vi "Trigger Level.vi"(7 "Read Value? (F)":bool, 8 "error in (no error)":errorcluster, 10 "Trigger Level (2.000 V)":dbl=2.0 min=-2.0 max=2.0 step=0.001 format="%.3g", 11 "VISA resource name":refnum<visa-resource-name>) -> (0 "error out":errorcluster, 2 "Trigger Level":dbl=2.0 format="%.3g", 3 "VISA resource name out":refnum<visa-resource-name>)   [LabVIEW 2013, in "SRS SR400.lvlib"]
doc: "<B>TL { v }</B>\n\nIf v is absent, the TL command returns the gate trigger level. When v is included, the trigger level is set to v Volts where -2.000 <= v <= 2.000. The resolution is .001 V."
uses:
  <instrlib>/SRS SR400/SRS SR400.lvlib
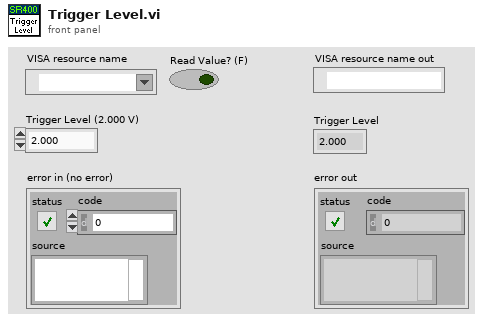
[diagram p1: front panel]
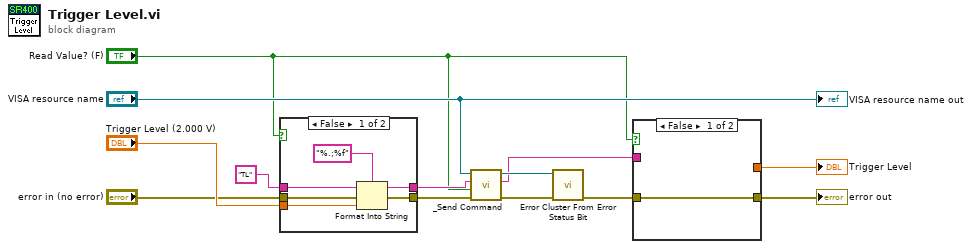
[diagram p0: block diagram]
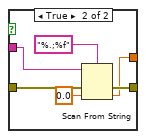
[diagram p2: hidden frame]
diagram:
  n1 = case shown="False" "Read Value? (F)" {
    tunnel: "Trigger Level (2.000 V)" -> [w19 _]
    tunnel: "error in (no error)" -> [w18 w20]
    tunnel: [w16 w21] -> w11
    tunnel: [w15 w20] -> w10
    tunnel: "TL" ("command") -> [w14 w21]
    frame False {
      n2 = Format Into String(format string="%.;%f", initial string=w14, error in=w18, w19) -> (resulting string=w16:string, error out=w15:errorcluster)
    }
    frame True {
    }
  }
  n3 = call <instrlib>:"_Send Command.vi"("error in (no error)"=w10, "Read Value? (F)"="Read Value? (F)", "Command"=w11, "VISA resource name"="VISA resource name") -> ("error out"=w7:errorcluster, "Response"=w3:string, "VISA resource name out"=w8:refnum<visa-resource-name>)  [unwired: 5 out]
  n4 = call <instrlib>:"Error Cluster From Error Status Bit.vi"("error in (no error)"=w7, "VISA resource name"=w8) -> ("error out"=w5:errorcluster)  [unwired: 8 in, 1 out]
  n5 = case shown="False" "Read Value? (F)" {
    tunnel: w5 -> [w22 w28]
    tunnel: [w22 w27] -> w4
    tunnel: w3 -> [_ w25]
    tunnel: [_ w23] -> w2
    frame False {
    }
    frame True {
      n6 = Scan From String(format string="%.;%f", input string=w25, error in=w28, default 1=0.0 ("default value 1")) -> (error out=w27:errorcluster, output 1=w23:dbl)  [unwired: 1 in, 2 out]
    }
  }
  "error out" <- w4
  "Trigger Level" <- w2
  "VISA resource name out" <- "VISA resource name"
